vi "Add To DAQmx Task.vi"(6 "Ignore Cal? (F)":bool, 7 "Frequency in":refnum<class "Frequency.lvclass">, 8 "error in (no error)":errorcluster, 9 "Scale Name":string, 10 "Chassis Name":string, 11 "task in":refnum<k21>) -> (0 "error out":errorcluster, 2 "Phys Chan Added":string, 3 "task out":refnum<k21>)   [LabVIEW 2012, in "Measurement Channels.lvlib" / "Frequency.lvclass"]
uses:
  Frequency.lvclass
  Class Channel/Read ChanName.vi
  Class Channel/Read Alias.vi
  Class Voltage/Read VRange.vi
  Class Voltage/Read Term Cfg.vi
  Class Voltage/Read Coupling.vi
  <vilib>/DAQmx/create/channels.llb/DAQmx Create Channel (AI-Voltage-Basic).vi
  <resource>/objmgr/daqmx.rc
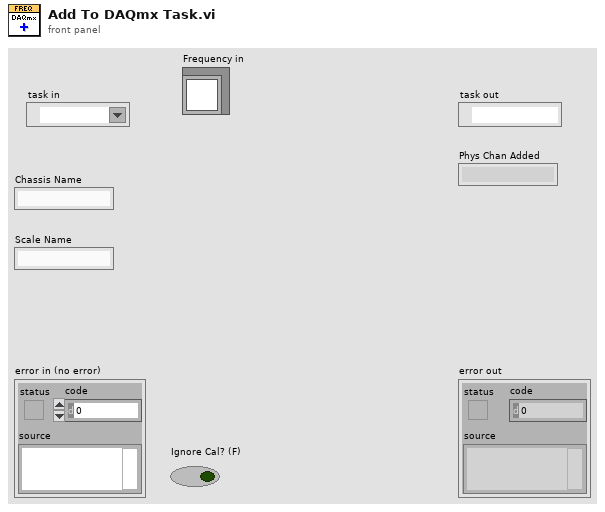
[diagram p1: front panel]
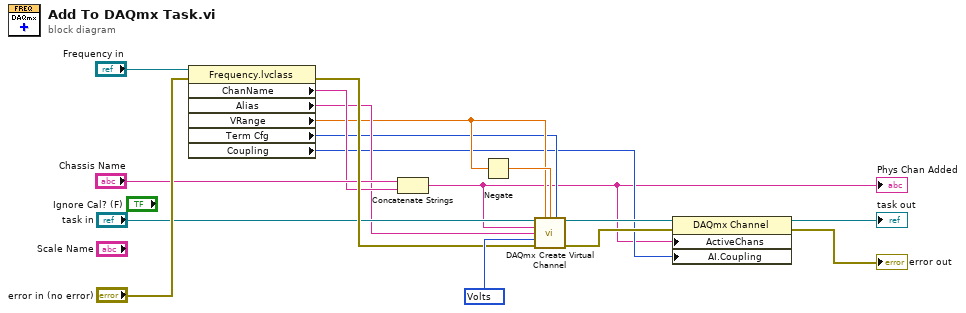
[diagram p0: block diagram]
diagram:
  w14 = 10348 items=["Volts"=10348, "From Custom Scale"=10065] ("units")
  n1 = property class="Frequency.lvclass"(reference="Frequency in", error in="error in (no error)") -> (error out=w11:errorcluster, "ChanName"=w8:string, "Alias"=w5:string, "VRange"=w4:dbl, "Term Cfg"=w3:u16, "Coupling"=w2:u16)  [unwired: 1 out]
  n2 = Concatenate Strings("Chassis Name", w8) -> (w1:string)
  "Phys Chan Added" <- w1
  n3 = Negate(x=w4) -> (-x=w13:dbl)
  n4 = call-poly <vilib>:"DAQmx Create Virtual Channel.vi"("task in"="task in", "maximum value"=w4, "minimum value"=w13, "input terminal configuration"=w3, "physical channels"=w1, "name to assign"=w5, "units"=w14, "error in"=w11) -> ("task out"=w15:refnum<k21>, "error out"=w16:errorcluster)  [unwired: 6 in]
  n5 = property class="DAQmx Channel"(reference=w15, error in=w16, "ActiveChans"=w1, "AI.Coupling"=w2) -> (reference out=→"task out":refnum<k21>, error out=→"error out":errorcluster)
